vi "Delete Reference.vi"(0 "all descendents":refnum<vi>[](array[refnum]), 5 "numeric":i32, 11 "error in":errorcluster) -> (15 "error out":errorcluster)   [LabVIEW 2021, in "Converter.lvlib"]
uses:
  Converter.lvlib
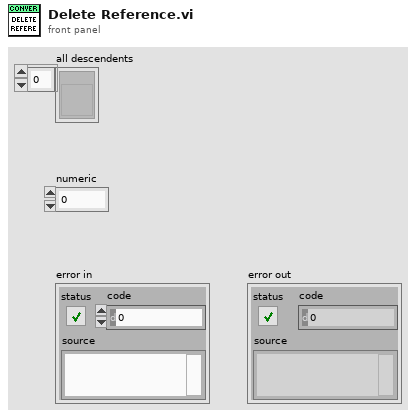
[diagram p1: front panel]
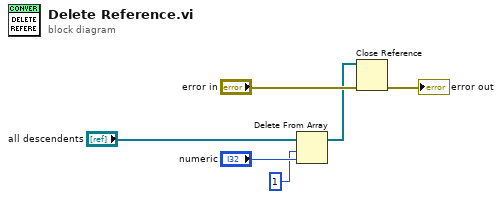
[diagram p0: block diagram]
diagram:
  n1 = Delete From Array(array="all descendents", length=1, index="numeric") -> (array with subset deleted=w4:refnum<vi>[])  [unwired: 1 out]
  n2 = Close Reference(reference=w4, error in (no error)="error in") -> (error out=→"error out":errorcluster)
